vi "_builtins_visibles_hide.vi"(8 "error in (no error)":errorcluster, 11 "GObjects in":refnum<vi>[](array[refnum])) -> (0 "error out":errorcluster, 2 "Reset Visible":T1(array[cluster]), 3 "GObjects out":refnum<vi>[](array[refnum]))   [LabVIEW 2019, in "Script.lvlib"]
doc: "Temporarily hide all display object connected to the GObject. \n\nCreated by: Ryan Pacini"
uses:
  Script.lvlib
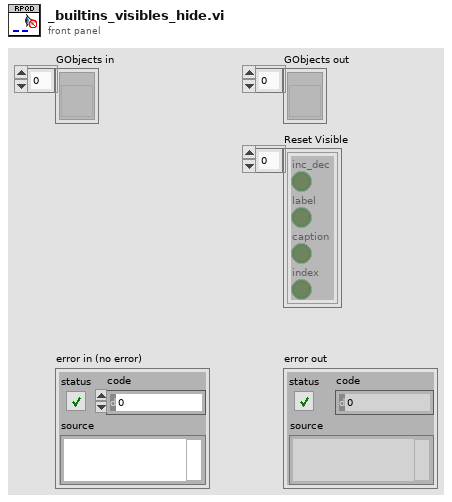
[diagram p1: front panel]
types:
  T1 = cluster{"inc_dec":bool, "label":bool, "caption":bool, "index":bool}[]
  T2 = cluster{"inc_dec":bool, "label":bool, "caption":bool, "index":bool}
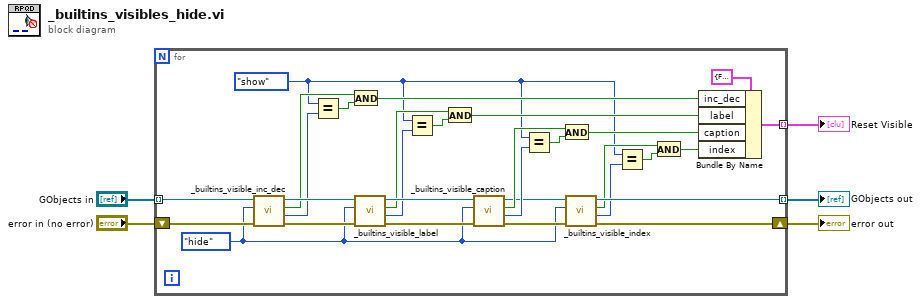
[diagram p0: block diagram]
diagram:
  n1 = for {
    tunnel: "GObjects in" -> [w34] mode=indexing
    shift-right: [w14] -> w3
    shift-left: "error in (no error)" -> [w35]
    tunnel: [w12] -> w2 mode=indexing
    tunnel: [w16] -> w1 mode=indexing
    w7 = enum8{"hide", "show"}."show" ("inc/dec")
    w10 = enum8{"hide", "show"}."hide" ("inc/dec")
    n2 = call "_builtins_visible_inc_dec.vi"("error in (no error)"=w35, "inc/dec"=w10, "GObject in"=w34) -> ("error out"=w30:errorcluster, "was inc/dec visible?"=w28:enum8{"hide", "show"}, "has inc/dec?"=w29:bool, "GObject out"=w31:refnum<vi>)  [unwired: 5 in]
    n3 = Equal?(x=w7, y=w28) -> (x = y?=w27:bool)
    n4 = And(x=w29, y=w27) -> (x .and. y?=w26:bool)
    n5 = call "_builtins_visible_label.vi"("error in (no error)"=w30, "label"=w10, "GObject in"=w31) -> ("error out"=w32:errorcluster, "was label visible?"=w23:enum8{"hide", "show"}, "has label?"=w24:bool, "GObject out"=w33:refnum<vi>)  [unwired: 5 in]
    n6 = Equal?(x=w7, y=w23) -> (x = y?=w25:bool)
    n7 = And(x=w24, y=w25) -> (x .and. y?=w22:bool)
    n8 = call "_builtins_visible_caption.vi"("error in (no error)"=w32, "caption"=w10, "GObject in"=w33) -> ("error out"=w15:errorcluster, "was caption visible?"=w19:enum8{"hide", "show"}, "has caption?"=w20:bool, "GObject out"=w13:refnum<vi>)  [unwired: 5 in]
    n9 = Equal?(x=w7, y=w19) -> (x = y?=w21:bool)
    n10 = And(x=w20, y=w21) -> (x .and. y?=w18:bool)
    n11 = call "_builtins_visible_index.vi"("error in (no error)"=w15, "index display"=w10, "GObject in"=w13) -> ("error out"=w14:errorcluster, "was index visible?"=w8:enum8{"hide", "show"}, "has index display?"=w9:bool, "GObject out"=w12:refnum<vi>)  [unwired: 5 in]
    n12 = Equal?(x=w7, y=w8) -> (x = y?=w11:bool)
    n13 = And(x=w9, y=w11) -> (x .and. y?=w6:bool)
    n14 = Bundle By Name(cluster=T2 {"inc_dec"=FALSE, "label"=FALSE, "caption"=FALSE, "index"=FALSE} ("reset"), "inc_dec"=w26, "label"=w22, "caption"=w18, "index"=w6) -> (w16:T2)
  }
  "GObjects out" <- w2
  "error out" <- w3
  "Reset Visible" <- w1
